vi "Template.Async.vi"(10 "Parameters":variant, 11 "Process":refnum<class "Process.lvclass">) -> ()   [LabVIEW 2026, in "NIDMM Engine.lvlib" / "NIDMM Engine.lvclass"]
uses:
  NIDMM Engine.lvclass
  NIDMM Engine.lvclass/NIDMM Engine.ctl
  <userlib>/NIVS Inline Async API (Express)/_Data Access Engine (Express)/Data Access Engine (Express)/Data Access Engine (Express).lvclass
  <userlib>/NIVS Inline Async API (Express)/_VS Inline Async API (Express)/Process/Process.lvclass
  Types/TargetSettings.ctl
  <vilib>/platform/TimedLoop/XDataNode/XDataNode.xnode
  <vilib>/Platform/TimedLoop/XDataNode/nitl_modes.ctl
  <vilib>/Platform/TimedLoop/XDataNode/XDNodeRunTimeDep.lvlib
  <vilib>/Platform/TimedLoop/XDataNode/wakeup.ctl
  <vilib>/Platform/TimedLoop/XDataNode/timing_clust.ctl
  <userlib>/NIVS Inline Async API (Express)/_Data Access Engine (Express)/Data Access Engine (Express)/Methods/Write.Lookup.vi
  <userlib>/NIVS Inline Async API (Express)/_Data Access Engine (Express)/Data Access Engine (Express)/Methods/Write.Data.vi
  <userlib>/NIVS Inline Async API (Express)/_Data Access Engine (Express)/Data Access Engine (Express)/Methods/Read.Lookup.vi
  <userlib>/NIVS Inline Async API (Express)/_Data Access Engine (Express)/Data Access Engine (Express)/Methods/Read.Data.vi
  <instrlib>/niDMM/nidmm.llb/niDMM Function.ctl
  Logging/Utilities/Log.Error.vi
  <instrlib>/niDMM/nidmm.llb/niDMM Configure Measurement Digits.vi
  Shared/CustomDeviceSettings.ctl
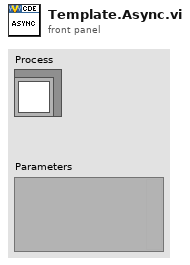
[diagram p1: front panel]
types:
  T1 = typedef "NIDMM Engine.lvlib/NIDMM Engine.lvclass/TargetSettings.ctl" = cluster{"instrument handle":refnum<k15>, "NIDMM":T2}
  T2 = typedef "CustomDeviceSettings.ctl" = cluster{"Name":string, "Properties":cluster{"ResourceName":string, "Model":string, "ScanPeriod(ms)":dbl, "ResolutionDigits":dbl, "ACMaxFrequency":dbl, "ACMinFrequency":dbl, "TargetOS":string, "TargetRate":dbl}, "Channels":cluster{"Mode[]":cluster{"Name":string, "DefaultValue":dbl, "Units":string, "GroupName":string, "Type":string, "Faultable":bool, "Scalable":bool, "ChannelDataReference":i32, "GroupIndex":i32}[], "ActiveMode[]":cluster{"Name":string, "DefaultValue":dbl, "Units":string, "GroupName":string, "Type":string, "Faultable":bool, "Scalable":bool, "ChannelDataReference":i32, "GroupIndex":i32}[], "DeviceStatus[]":cluster{"Name":string, "DefaultValue":dbl, "Units":string, "GroupName":string, "Type":string, "Faultable":bool, "Scalable":bool, "ChannelDataReference":i32, "GroupIndex":i32}[], "Heartbeat[]":cluster{"Name":string, "DefaultValue":dbl, "Units":string, "GroupName":string, "Type":string, "Faultable":bool, "Scalable":bool, "ChannelDataReference":i32, "GroupIndex":i32}[]}, "Sections":cluster{"Voltage[]":cluster{"Name":string, "Channels":cluster{"VoltageReading[]":cluster{"Name":string, "DefaultValue":dbl, "Units":string, "GroupName":string, "Type":string, "Faultable":bool, "Scalable":bool, "ChannelDataReference":i32, "GroupIndex":i32}[], "VoltageStatus[]":cluster{"Name":string, "DefaultValue":dbl, "Units":string, "GroupName":string, "Type":string, "Faultable":bool, "Scalable":bool, "ChannelDataReference":i32, "GroupIndex":i32}[], "VoltageFunction[]":cluster{"Name":string, "DefaultValue":dbl, "Units":string, "GroupName":string, "Type":string, "Faultable":bool, "Scalable":bool, "ChannelDataReference":i32, "GroupIndex":i32}[], "VoltageActualRange[]":cluster{"Name":string, "DefaultValue":dbl, "Units":string, "GroupName":string, "Type":string, "Faultable":bool, "Scalable":bool, "ChannelDataReference":i32, "GroupIndex":i32}[], "VoltageRange[]":cluster{"Name":string, "DefaultValue":dbl, "Units":string, "GroupName":string, "Type":string, "Faultable":bool, "Scalable":bool, "ChannelDataReference":i32, "GroupIndex":i32}[]}}[], "Current[]":cluster{"Name":string, "Channels":cluster{"CurrentReading[]":cluster{"Name":string, "DefaultValue":dbl, "Units":string, "GroupName":string, "Type":string, "Faultable":bool, "Scalable":bool, "ChannelDataReference":i32, "GroupIndex":i32}[], "CurrentStatus[]":cluster{"Name":string, "DefaultValue":dbl, "Units":string, "GroupName":string, "Type":string, "Faultable":bool, "Scalable":bool, "ChannelDataReference":i32, "GroupIndex":i32}[], "CurrentFunction[]":cluster{"Name":string, "DefaultValue":dbl, "Units":string, "GroupName":string, "Type":string, "Faultable":bool, "Scalable":bool, "ChannelDataReference":i32, "GroupIndex":i32}[], "CurrentActualRange[]":cluster{"Name":string, "DefaultValue":dbl, "Units":string, "GroupName":string, "Type":string, "Faultable":bool, "Scalable":bool, "ChannelDataReference":i32, "GroupIndex":i32}[], "CurrentRange[]":cluster{"Name":string, "DefaultValue":dbl, "Units":string, "GroupName":string, "Type":string, "Faultable":bool, "Scalable":bool, "ChannelDataReference":i32, "GroupIndex":i32}[]}}[]}}
  T3 = typedef "Data Access Engine (Express).lvlib/Data Access Engine (Express).lvclass/Write.DVR.ctl" = refnum<data-value>
  T4 = typedef "Data Access Engine (Express).lvlib/Data Access Engine (Express).lvclass/Read.DVR.ctl" = refnum<data-value>
  T5 = typedef "XDNodeRunTimeDep.lvlib/timing_clust.ctl" = cluster{"Expected End [f-1]":u64, "Actual End [f-1]":u64, "Finished Late? [f-1]":bool, "Expected End [i-1]":u64, "Actual End [i-1]":u64, "Finished Late? [i-1]":bool, "Expected Start [i]":u64, "Actual Start [i]":u64, "Expected Start [f]":u64, "Actual Start [f]":u64, "Source Name":string, "Structure Name":string, "Period":i64, "Deadline":i64, "Offset":i64, "Start":i64, "Priority":i32, "Timeout":i32, "Mode":T6, "Wakeup Reason":T7, "Error":errorcluster, "Source Type":string, "Secondary Source Type":string, "Global End Time":u64, "Global Start Time":u64, "Frame Duration":u64, "Iteration Duration":u64, "Assigned CPU":i32, "I/O Scan Engine Mode":u32}
  T6 = typedef "XDNodeRunTimeDep.lvlib/nitl_modes.ctl" = enum32{"No Change", "Process missed periods, maintain original phase", "Discard missed periods, maintain original phase", "Process missed periods, ignore original phase", "Discard missed periods, ignore original phase"}
  T7 = typedef "XDNodeRunTimeDep.lvlib/wakeup.ctl" = enum32{"Normal", "Aborted", "Asynchronous wakeup", "Timing source error", "Timed loop error", "Timeout"}
  T8 = typedef "niDMM Function.ctl" = enum16{"DC Volts", "AC Volts", "DC Current", "AC Current", "2-wire Resistance", "4-wire Resistance", "Diode", "Frequency", "Period", "AC Volts DC Coupled", "Capacitance", "Inductance", "Temperature"}
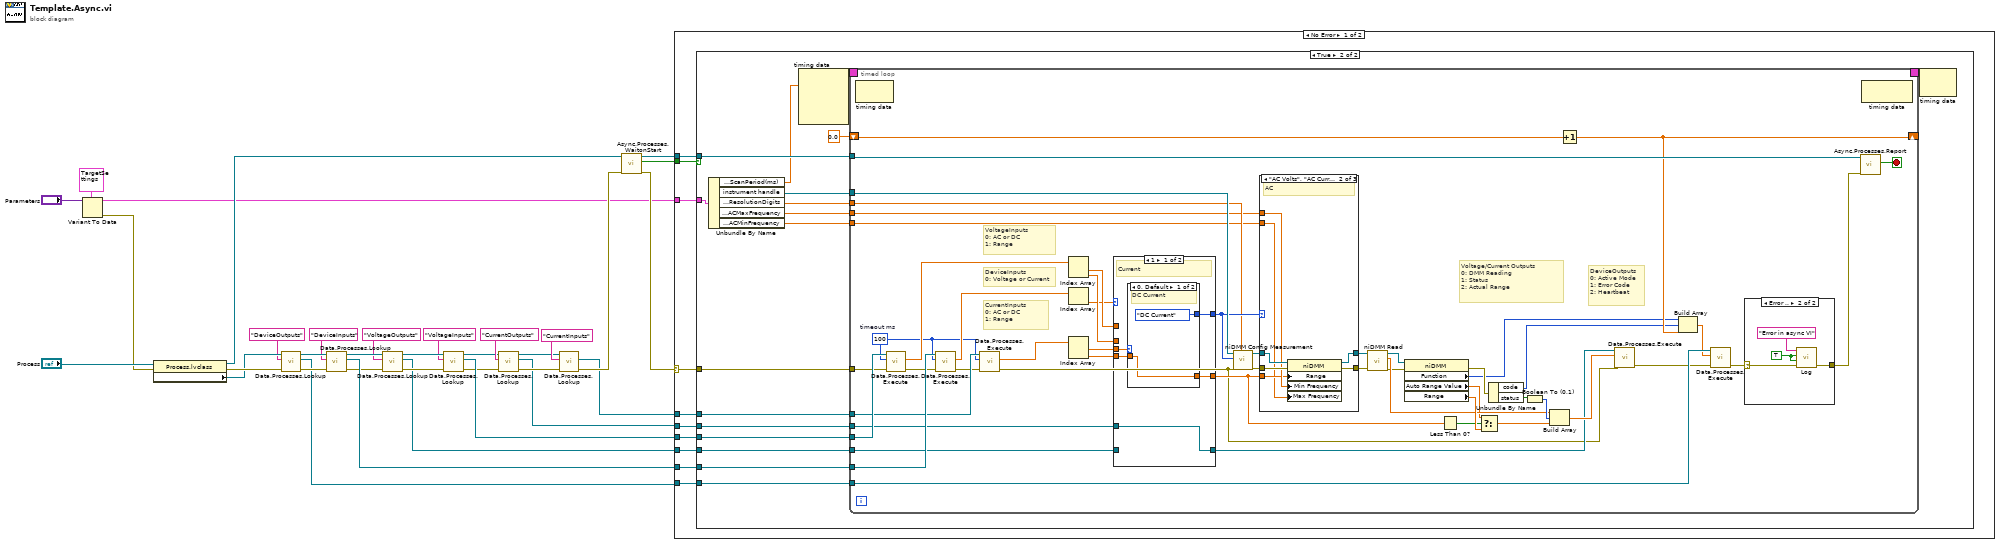
[diagram p0: block diagram]
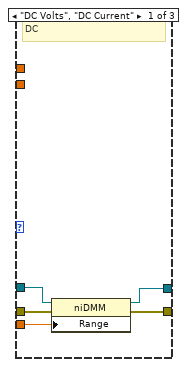
[diagram p3: hidden frame]
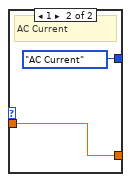
[diagram p6: hidden frame]
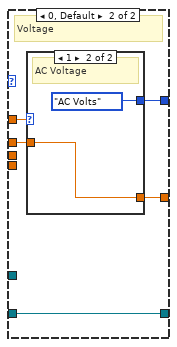
[diagram p7: hidden frame]
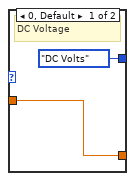
[diagram p8: hidden frame]
diagram:
  n1 = Variant To Data(type=T1 {"instrument handle"="Dev1", "NIDMM"={"Name"="", "Properties"={"ResourceName"="", "Model"="", "ScanPeriod(ms)"=0.0, "ResolutionDigits"=0.0, "ACMaxFrequency"=0.0, "ACMinFrequency"=0.0, "TargetOS"="", "TargetRate"=0.0}, "Channels"={"Mode[]"=[], "ActiveMode[]"=[], "DeviceStatus[]"=[], "Heartbeat[]"=[]}, "Sections"={"Voltage[]"=[], "Current[]"=[]}}} ("Target Settings"), Variant="Parameters") -> (data=w2:T1, error out=w1:errorcluster)  [unwired: 1 in]
  n2 = property class="Process.lvclass"(reference="Process", error in=w1) -> (reference out=w28:refnum<class "Process.lvclass">, error out=w32:errorcluster, "Data Member Access:Data Access"=w30:refnum<class "Data Access Engine (Express).lvclass">)
  n3 = call-poly <userlib>:"Data.Processes.Lookup.vi"("error in"=w32, "Name"="DeviceOutputs", "Data Access API in"=w30) -> ("error out"=w33:errorcluster, "Ref"=w25:T3, "Data Access API out"=w29:refnum<class "Data Access Engine (Express).lvclass">)  [unwired: 5 in, 1 out]
  n4 = call-poly <userlib>:"Data.Processes.Lookup.vi"("error in"=w33, "Name"="DeviceInputs", "Data Access API in"=w29) -> ("error out"=w4:errorcluster, "Ref"=w26:T4, "Data Access API out"=w18:refnum<class "Data Access Engine (Express).lvclass">)  [unwired: 5 in, 1 out]
  n5 = call-poly <userlib>:"Data.Processes.Lookup.vi"("error in"=w4, "Name"="VoltageOutputs", "Data Access API in"=w18) -> ("error out"=w17:errorcluster, "Ref"=w6:T3, "Data Access API out"=w19:refnum<class "Data Access Engine (Express).lvclass">)  [unwired: 5 in, 1 out]
  n6 = call-poly <userlib>:"Data.Processes.Lookup.vi"("error in"=w17, "Name"="VoltageInputs", "Data Access API in"=w19) -> ("error out"=w13:errorcluster, "Ref"=w15:T4, "Data Access API out"=w9:refnum<class "Data Access Engine (Express).lvclass">)  [unwired: 5 in, 1 out]
  n7 = call-poly <userlib>:"Data.Processes.Lookup.vi"("error in"=w13, "Name"="CurrentOutputs", "Data Access API in"=w9) -> ("error out"=w14:errorcluster, "Ref"=w7:T3, "Data Access API out"=w8:refnum<class "Data Access Engine (Express).lvclass">)  [unwired: 5 in, 1 out]
  n8 = call-poly <userlib>:"Data.Processes.Lookup.vi"("error in"=w14, "Name"="CurrentInputs", "Data Access API in"=w8) -> ("error out"=w10:errorcluster, "Ref"=w3:T4)  [unwired: 5 in, 2 out]
  n9 = call <userlib>:"Async.Processes.WaitonStart.vi"("error in"=w10, "Process in"=w28) -> ("error out"=w34:errorcluster, "Execute"=w27:bool, "Process out"=w24:refnum<class "Process.lvclass">)  [unwired: 7 in]
  n10 = case shown="No Error" w34 {
    selector: w34 -> [w44 _]
    tunnel: w27 -> [w43 _]
    tunnel: w26 -> [w42 _]
    tunnel: w25 -> [w41 _]
    tunnel: w24 -> [w40 _]
    tunnel: w6 -> [w39 _]
    tunnel: w15 -> [w38 _]
    tunnel: w7 -> [w37 _]
    tunnel: w3 -> [w36 _]
    tunnel: w2 -> [w35 _]
    frame No Error {
      n11 = case shown="True" w43 {
        tunnel: w44 -> [_ w61]
        tunnel: w42 -> [_ w51]
        tunnel: w41 -> [_ w60]
        tunnel: w40 -> [_ w59]
        tunnel: w39 -> [_ w55]
        tunnel: w38 -> [_ w54]
        tunnel: w37 -> [_ w53]
        tunnel: w36 -> [_ w52]
        tunnel: w35 -> [_ w50]
        frame False {
        }
        frame True {
          n12 = Unbundle By Name(w50) -> ("NIDMM.Properties.ScanPeriod(ms)"=w48:dbl, "instrument handle"=w49:refnum<k15>, "NIDMM.Properties.ResolutionDigits"=w47:dbl, "NIDMM.Properties.ACMaxFrequency"=w46:dbl, "NIDMM.Properties.ACMinFrequency"=w45:dbl)
          n13 = node-c288(w48) -> (w58:T5)  [unwired: 3 in]
          n14 = timed-loop {
            tunnel: w61 -> [w100]
            tunnel: w51 -> [w112]
            tunnel: w60 -> [w111]
            tunnel: w59 -> [w110]
            timing: w58 -> [_]
            timing-out: [_] -> w57
            shift-right: [w105] -> _
            shift-left: 0.0 -> [w107]
            tunnel: w55 -> [w104]
            tunnel: w54 -> [w101]
            tunnel: w53 -> [w93]
            tunnel: w52 -> [w95]
            tunnel: w46 -> [w69]
            tunnel: w49 -> [w90]
            tunnel: w47 -> [w70]
            tunnel: w45 -> [w68]
            stop <- w109 stop-if-true
            w72 = 100  # timeout ms
            # "DeviceOutputs\n0: Active Mode\n1: Error Code\n2: Heartbeat"
            # "Voltage/Current Outputs\n0: DMM Reading\n1: Status\n2: Actual Range"
            # "CurrentInputs\n0: AC or DC\n1: Range"
            # "DeviceInputs\n0: Voltage or Current"
            # "VoltageInputs\n0: AC or DC\n1: Range"
            n15 = node-c288() -> ()  [unwired: 1 in, 1 out]
            n16 = call-poly <userlib>:"Data.Processes.Execute.vi"("error in"=w100, "timeout ms"=w72, "Ref"=w101) -> ("error out"=w99:errorcluster, "Values"=w98:dbl[])  [unwired: 6 in, 1 out]
            n17 = call-poly <userlib>:"Data.Processes.Execute.vi"("error in"=w99, "timeout ms"=w72, "Ref"=w112) -> ("error out"=w94:errorcluster, "Values"=w108:dbl[])  [unwired: 6 in, 1 out]
            n18 = call-poly <userlib>:"Data.Processes.Execute.vi"("error in"=w94, "timeout ms"=w72, "Ref"=w95) -> ("error out"=w67:errorcluster, "Values"=w96:dbl[])  [unwired: 6 in, 1 out]
            n19 = Index Array(array=w98) -> (element #1=w89:dbl, element #2=w97:dbl)  [unwired: 2 in]
            n20 = Index Array(array=w108) -> (element=w63:dbl)  [unwired: 1 in]
            n21 = Index Array(array=w96) -> (element #1=w91:dbl, element #2=w92:dbl)  [unwired: 2 in]
            n22 = case shown="1" w63 {
              tunnel: w89 -> [_ w147]
              tunnel: [w138 w146] -> w87
              tunnel: w97 -> [_ w145]
              tunnel: [w137 w144] -> w74
              tunnel: w92 -> [w136 _]
              tunnel: [w135 w143] -> w73
              tunnel: w104 -> [_ w143]
              tunnel: w93 -> [w135 _]
              tunnel: w91 -> [w134 _]
              frame 1 {
                # "Current"
                n23 = case shown="0, Default" w134 {
                  tunnel: [niDMM_Function."DC Current" ("Function") niDMM_Function."AC Current" ("Function")] -> w138
                  tunnel: [w139 w141] -> w137
                  tunnel: w136 -> [w139 w141]
                  frame 0, Default {
                    # "DC Current"
                  }
                  frame 1 {
                    # "AC Current"
                  }
                }
              }
              frame 0, Default {
                # "Voltage"
                n24 = case shown="1" w147 {
                  tunnel: [niDMM_Function."DC Volts" ("Function") niDMM_Function."AC Volts" ("Function")] -> w146
                  tunnel: w145 -> [w148 w150]
                  tunnel: [w148 w150] -> w144
                  frame 0, Default {
                    # "DC Voltage"
                  }
                  frame 1 {
                    # "AC Voltage"
                  }
                }
              }
            }
            n25 = call-poly <instrlib>:"niDMM Config Measurement.vi"("Resolution in Digits"=w70, "error in (no error)"=w67, "Function"=w87, "instrument handle"=w90) -> ("error out"=w88:errorcluster, "instrument handle out"=w86:refnum<k15>)  [unwired: 6 in]
            n26 = case shown="\"AC Volts\", \"AC Current\"" w87 {
              tunnel: w88 -> [w117 w124 w125]
              tunnel: w86 -> [w115 w123 w126]
              tunnel: [w116 w122 w125] -> w76
              tunnel: [w114 w121 w126] -> w75
              tunnel: w74 -> [w113 w119 _]
              tunnel: w69 -> [_ w120 _]
              tunnel: w68 -> [_ w118 _]
              frame "DC Volts", "DC Current" {
                # "DC"
                n27 = property class="niDMM"(reference=w115, error in=w117, "Range"=w113) -> (reference out=w114:refnum<k15>, error out=w116:errorcluster)
              }
              frame "AC Volts", "AC Current" {
                # "AC"
                n28 = property class="niDMM"(reference=w123, error in=w124, "Range"=w119, "Min Frequency"=w120, "Max Frequency"=w118) -> (reference out=w121:refnum<k15>, error out=w122:errorcluster)
              }
              frame Default {
              }
            }
            n29 = call <instrlib>:"niDMM Read.vi"("error in (no error)"=w76, "instrument handle"=w75) -> ("error out"=w78:errorcluster, "Measurement"=w79:dbl, "instrument handle out"=w77:refnum<k15>)  [unwired: 7 in]
            n30 = property class="niDMM"(reference=w77, error in=w78) -> (error out=w66:errorcluster, "Function"=w62:i32, "Auto Range Value"=w64:dbl, "Range"=w84:dbl)  [unwired: 1 out]
            n31 = Less Than 0?(x=w74) -> (x < 0?=w83:bool)
            n32 = Select(t=w64, s=w83, f=w84) -> (s? t:f=w85:dbl)
            n33 = Unbundle By Name(w66) -> ("code"=w65:i32, "status"=w81:bool)
            n34 = Boolean To (0,1)(Boolean=w81) -> (0, 1=w82:i16)
            n35 = Build Array(w79, w82, w85) -> (w80:dbl[])
            n36 = Increment(x=w107) -> (x+1=w105:dbl)
            n37 = call-poly <userlib>:"Data.Processes.Execute.vi"("error in"=w67, "Values"=w80, "Ref"=w73) -> ("error out"=w71:errorcluster)  [unwired: 8 in]
            n38 = Build Array(w62, w65, w105) -> (w106:dbl[])
            n39 = call-poly <userlib>:"Data.Processes.Execute.vi"("error in"=w71, "Values"=w106, "Ref"=w111) -> ("error out"=w103:errorcluster)  [unwired: 8 in]
            n40 = case shown="Error .." w103 {
              selector: w103 -> [w129 w132]
              tunnel: [w129 w131] -> w102
              frame No Error {
              }
              frame Error {
                w130 = TRUE ("Add to log file? (F)")
                n41 = call-poly "Log.vi"("error in"=w132, "Append newline? (T)"=w130, "Add to log file? (F)"=w130, "Message"="Error in async VI") -> ("error out"=w131:errorcluster)  [unwired: 7 in]
              }
            }
            n42 = call <userlib>:"Async.Processes.Report.vi"("error in"=w102, "Process in"=w110) -> ("Stop"=w109:bool)  [unwired: 8 in, 1 out]
            n43 = node-c288() -> ()  [unwired: 1 in, 1 out]
          }
          n44 = node-c288(w57) -> ()  [unwired: 1 out]
        }
      }
    }
    frame Error {
    }
  }
